vi "Autonomous Independent.vi"() -> ()   [LabVIEW 2016]
doc: "This VI is called when autonomous begins, and will automatically be terminated when autonomous ends. You can carry out timed or sensor driven robot movement independently without needing to return to the caller."
uses:
  2_8_17/Auto_Action.ctl
  <vilib>/Rock Robotics/Network Tables/NT Read Number.vi
  2_11_17/Systems/Global 1.vi
panel:
  out "Auto Mode":dbl=7.0
  in  "Auton_Modes":T2(array[cluster])=[{"Actions"=[{"Effort"=0.55, "Duration"=3.5, "Action"=enum."Nothing", "Encoder"=0.0, "Condition"=FALSE}, {"Effort"=0.0, "Duration"=0.0, "Action"=enum."Nothing", "Encoder"=0.0, "Condition"=FALSE}]}, {"Actions"=[{"Effort"=0.0, "Duration"=0.1, "Action"=enum."Gear1", "Encoder"=6.462, "Condition"=FALSE}, {"Effort"=0.0, "Duration"=0.1, "Action"=enum."Nothing", "Encoder"=0.0, "Condition"=FALSE}, {"Effort"=0.25, "Duration"=1.0, "Action"=enum."Nothing", "Encoder"=38.0, "Condition"=FALSE}, {"Effort"=0.0, "Duration"=0.1, "Action"=enum."Nothing", "Encoder"=0.0, "Condition"=FALSE}, {"Effort"=0.25, "Duration"=0.0, "Action"=enum."Nothing", "Encoder"=57.0, "Condition"=FALSE}, {"Effort"=-0.25, "Duration"=0.0, "Action"=enum."Nothing", "Encoder"=0.0, "Condition"=FALSE}, {"Effort"=1.0, "Duration"=0.0, "Action"=enum."Nothing", "Encoder"=0.0, "Condition"=FALSE}, {"Effort"=0.25, "Duration"=0.0, "Action"=enum."Nothing", "Encoder"=0.0, "Condition"=FALSE}]}, {"Actions"=[{"Effort"=0.0, "Duration"=0.1, "Action"=enum."Drive Encoder Reset", "Encoder"=0.0, "Condition"=FALSE}, {"Effort"=0.0, "Duration"=1.0, "Action"=enum."Gyro Reset", "Encoder"=0.0, "Condition"=FALSE}, {"Effort"=0.3, "Duration"=2.0, "Action"=enum."Drive", "Encoder"=88.0, "Condition"=TRUE}, {"Effort"=1.0, "Duration"=1.0, "Action"=enum."Gear0", "Encoder"=0.0, "Condition"=FALSE}, {"Effort"=1.0, "Duration"=1.0, "Action"=enum."Gear0", "Encoder"=0.0, "Condition"=FALSE}, {"Effort"=1.0, "Duration"=0.5, "Action"=enum."Nothing", "Encoder"=0.0, "Condition"=FALSE}, {"Effort"=0.0, "Duration"=0.0, "Action"=enum."Drive Encoder Reset", "Encoder"=0.0, "Condition"=FALSE}, {"Effort"=0.3, "Duration"=0.5, "Action"=enum."Nothing", "Encoder"=24.0, "Condition"=TRUE}, {"Effort"=0.0, "Duration"=0.0, "Action"=enum."Nothing", "Encoder"=0.0, "Condition"=FALSE}, {"Effort"=-0.2, "Duration"=0.75, "Action"=enum."Drive", "Encoder"=24.0, "Condition"=FALSE}, {"Effort"=0.0, "Duration"=0.0, "Action"=enum."Drive Encoder Reset", "Encoder"=0.0, "Condition"=FALSE}, {"Effort"=-0.25, "Duration"=0.0, "Action"=enum."Nothing", "Encoder"=12.0, "Condition"=FALSE}]}, {"Actions"=[{"Effort"=0.0, "Duration"=0.1, "Action"=enum."Drive Encoder Reset", "Encoder"=6.462, "Condition"=FALSE}, {"Effort"=0.0, "Duration"=0.1, "Action"=enum."Gyro Reset", "Encoder"=0.0, "Condition"=FALSE}, {"Effort"=-0.25, "Duration"=1.0, "Action"=enum."Drive", "Encoder"=6.462, "Condition"=FALSE}, {"Effort"=0.0, "Duration"=0.1, "Action"=enum."Gyro Reset", "Encoder"=0.0, "Condition"=FALSE}, {"Effort"=-0.25, "Duration"=0.0, "Action"=enum."Turn", "Encoder"=57.0, "Condition"=FALSE}, {"Effort"=-0.25, "Duration"=0.0, "Action"=enum."Drive", "Encoder"=7.5, "Condition"=FALSE}, {"Effort"=-1.0, "Duration"=0.0, "Action"=enum."Gear0", "Encoder"=0.0, "Condition"=FALSE}, {"Effort"=0.25, "Duration"=0.0, "Action"=enum."Drive", "Encoder"=3.0, "Condition"=FALSE}]}, {"Actions"=[{"Effort"=0.0, "Duration"=0.1, "Action"=enum."Drive Encoder Reset", "Encoder"=6.462, "Condition"=FALSE}, {"Effort"=0.0, "Duration"=0.1, "Action"=enum."Gyro Reset", "Encoder"=0.0, "Condition"=FALSE}, {"Effort"=-0.25, "Duration"=1.0, "Action"=enum."Drive", "Encoder"=6.462, "Condition"=FALSE}, {"Effort"=0.0, "Duration"=0.1, "Action"=enum."Gyro Reset", "Encoder"=0.0, "Condition"=FALSE}, {"Effort"=-0.25, "Duration"=0.0, "Action"=enum."Turn", "Encoder"=57.0, "Condition"=FALSE}, {"Effort"=-0.25, "Duration"=0.0, "Action"=enum."Drive", "Encoder"=7.5, "Condition"=FALSE}, {"Effort"=-1.0, "Duration"=0.0, "Action"=enum."Gear0", "Encoder"=0.0, "Condition"=FALSE}, {"Effort"=0.25, "Duration"=0.0, "Action"=enum."Drive", "Encoder"=3.0, "Condition"=FALSE}]}, {"Actions"=[{"Effort"=0.0, "Duration"=0.1, "Action"=enum."Drive Encoder Reset", "Encoder"=0.0, "Condition"=FALSE}, {"Effort"=0.0, "Duration"=0.1, "Action"=enum."Gyro Reset", "Encoder"=0.0, "Condition"=FALSE}, {"Effort"=0.25, "Duration"=1.0, "Action"=enum."Drive", "Encoder"=6.462, "Condition"=FALSE}, {"Effort"=1.0, "Duration"=0.1, "Action"=enum."Gyro Reset", "Encoder"=0.0, "Condition"=FALSE}, {"Effort"=0.25, "Duration"=0.0, "Action"=enum."Turn", "Encoder"=57.0, "Condition"=FALSE}, {"Effort"=0.25, "Duration"=0.0, "Action"=enum."Drive", "Encoder"=7.5, "Condition"=FALSE}, {"Effort"=1.0, "Duration"=0.0, "Action"=enum."Gear0", "Encoder"=0.0, "Condition"=FALSE}, {"Effort"=-0.25, "Duration"=0.0, "Action"=enum."Drive", "Encoder"=3.0, "Condition"=FALSE}]}, {"Actions"=[{"Effort"=0.0, "Duration"=0.1, "Action"=enum."Drive Encoder Reset", "Encoder"=0.0, "Condition"=FALSE}, {"Effort"=0.0, "Duration"=0.1, "Action"=enum."Gyro Reset", "Encoder"=0.0, "Condition"=FALSE}, {"Effort"=0.25, "Duration"=5.0, "Action"=enum."Drive", "Encoder"=60000.0, "Condition"=TRUE}, {"Effort"=0.75, "Duration"=1.0, "Action"=enum."Nothing", "Encoder"=0.0, "Condition"=FALSE}, {"Effort"=0.0, "Duration"=1.0, "Action"=enum."Nothing", "Encoder"=0.0, "Condition"=FALSE}, {"Effort"=0.0, "Duration"=0.0, "Action"=enum."Nothing", "Encoder"=0.0, "Condition"=FALSE}]}, {"Actions"=[{"Effort"=0.0, "Duration"=0.5, "Action"=enum."Drive Encoder Reset", "Encoder"=0.0, "Condition"=FALSE}, {"Effort"=0.55, "Duration"=4.25, "Action"=enum."Gyro Reset", "Encoder"=0.0, "Condition"=FALSE}, {"Effort"=0.3, "Duration"=0.0, "Action"=enum."Drive", "Encoder"=60.0, "Condition"=FALSE}, {"Effort"=0.25, "Duration"=1.5, "Action"=enum."Turn", "Encoder"=0.0, "Condition"=FALSE}, {"Effort"=0.25, "Duration"=2.0, "Action"=enum."Vision Correction", "Encoder"=76.6, "Condition"=FALSE}, {"Effort"=0.3, "Duration"=0.5, "Action"=enum."Drive", "Encoder"=0.0, "Condition"=TRUE}]}, {"Actions"=[{"Effort"=0.0, "Duration"=0.0, "Action"=enum."Nothing", "Encoder"=0.0, "Condition"=FALSE}]}]
  # "Nothing"
  # "Boiler Right Right side gear"
  # "Middle Gear"
  # "Boiler Right Left Side Gear"
  # "Boiler Left RightSide Gear"
  # "Boiler Left Left Side Gear"
  # "Drive"
  # "Vision Correction"
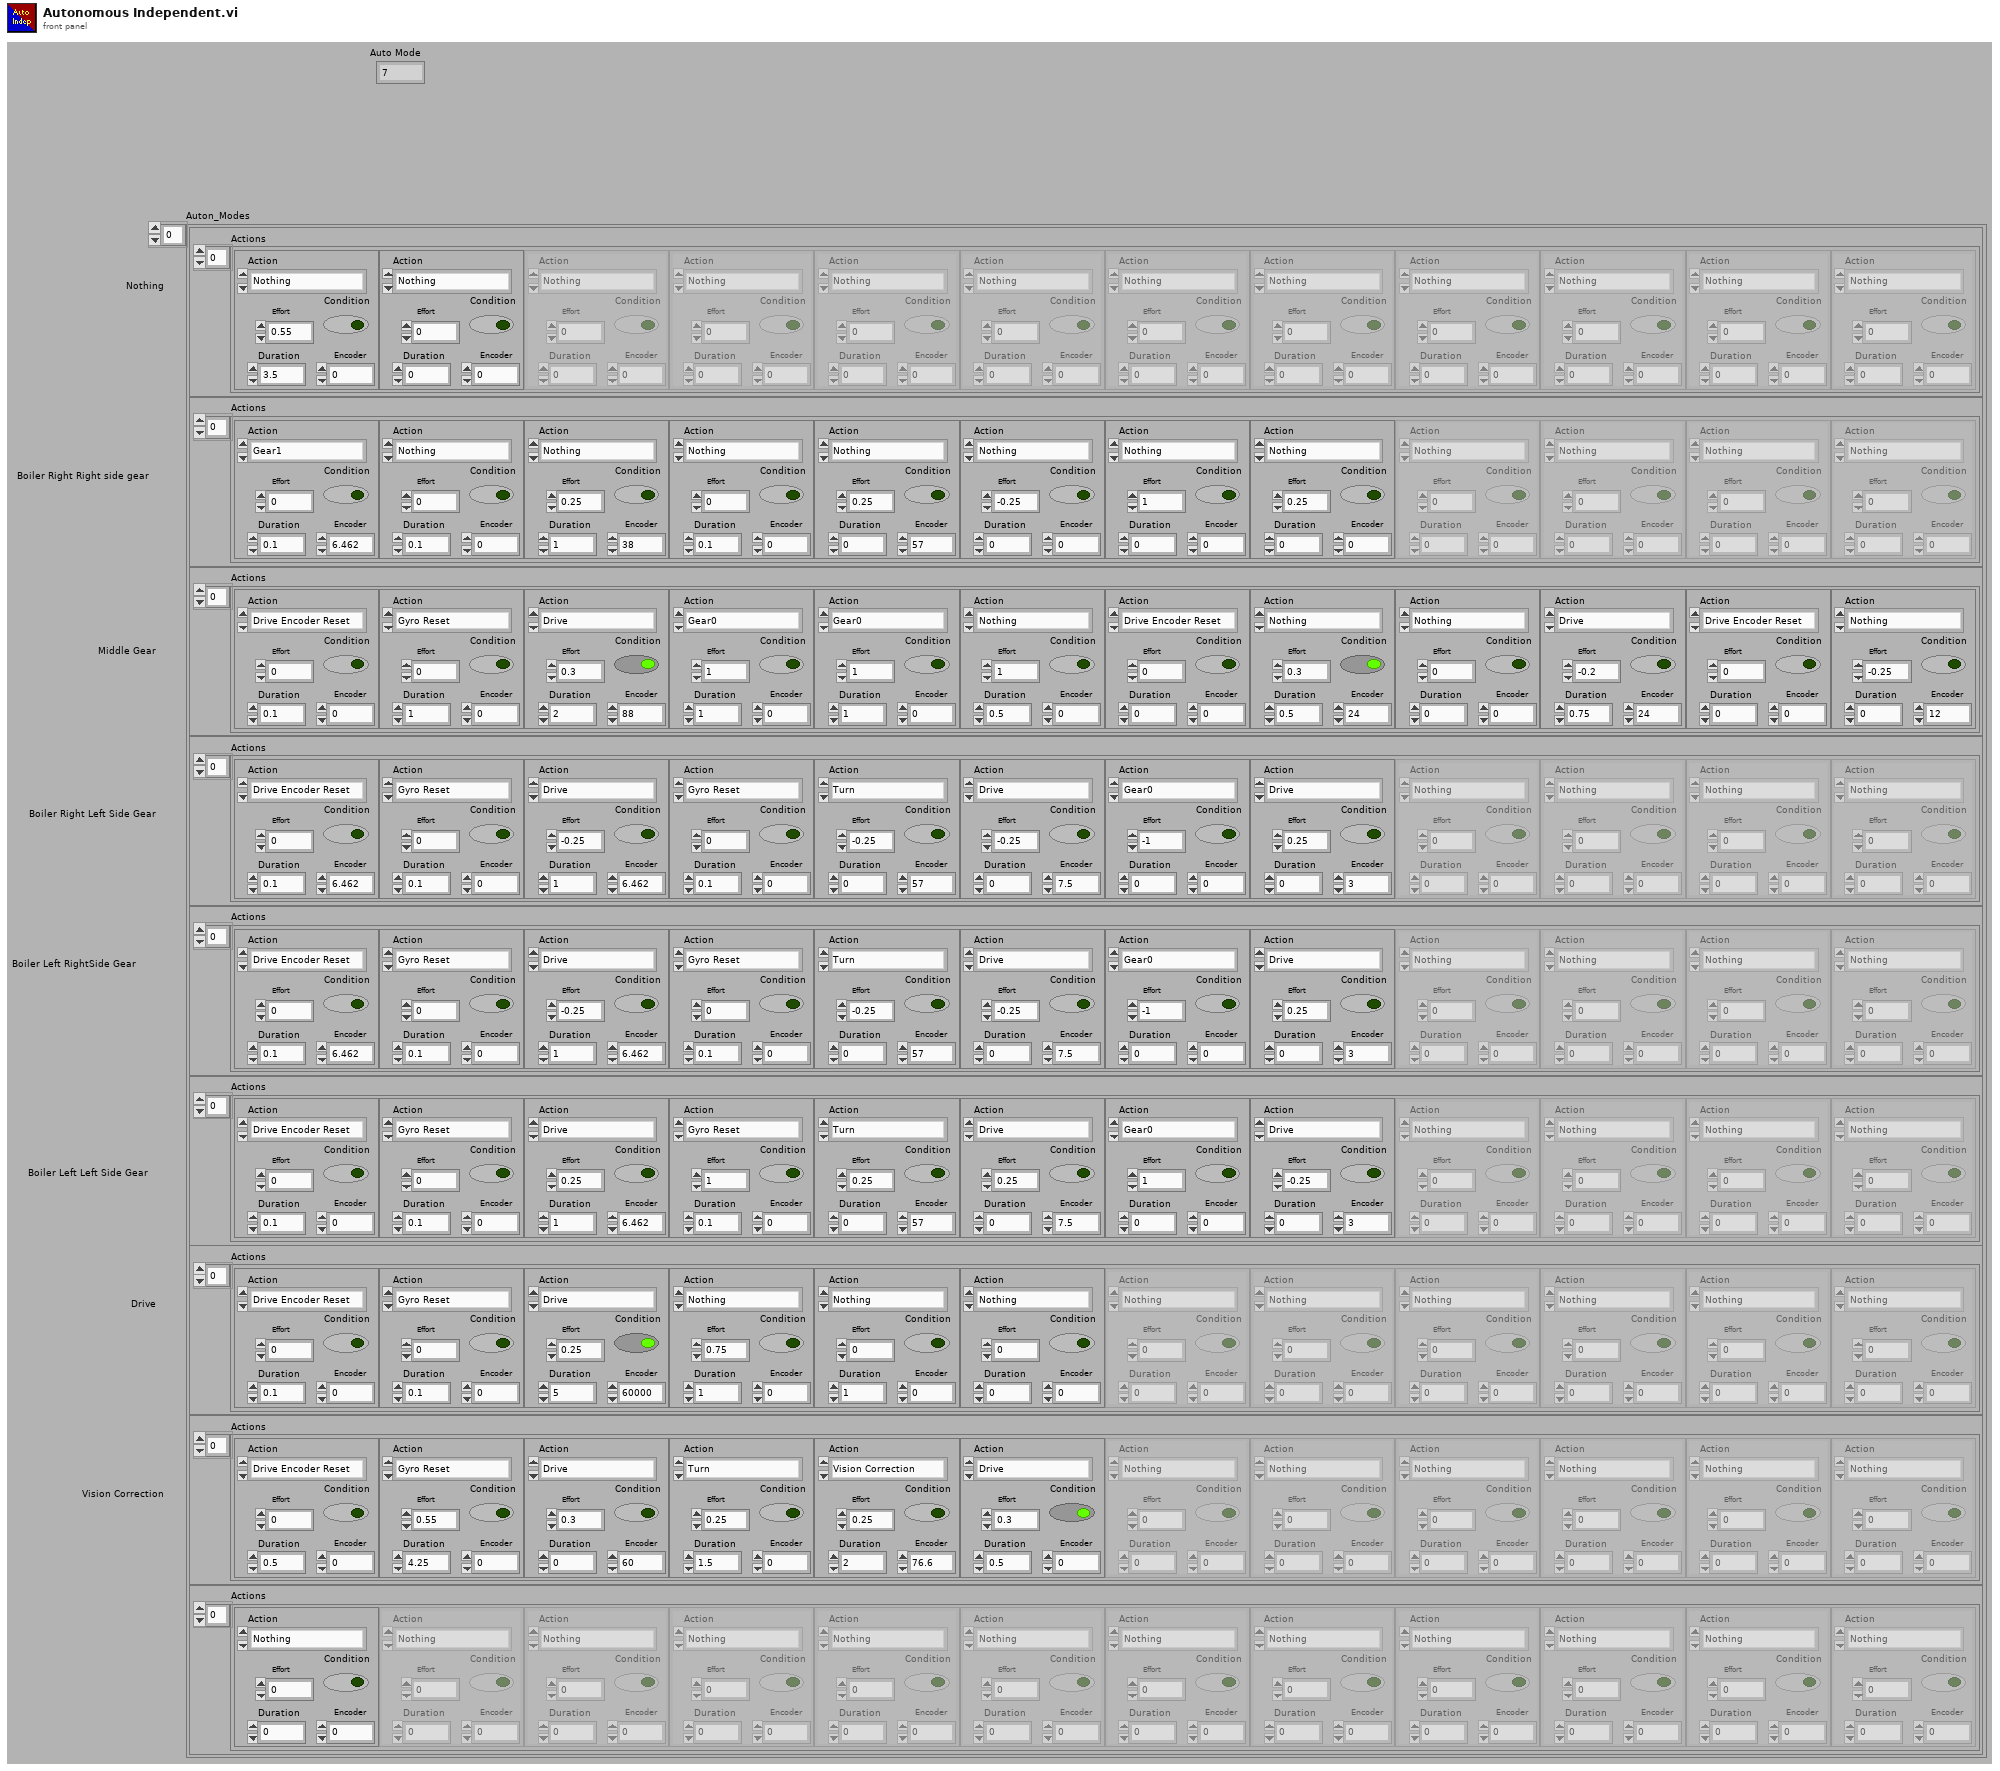
[diagram p1: front panel]
types:
  T1 = typedef "Auto_Action.ctl" = enum16{"Nothing", "Drive", "Vision Correction", "Turn", "Gear0", "Gear1", "Climb", "Intake", "Index", "Shoot", "Test", "Drive Encoder Reset", "Gyro Reset"}
  T2 = cluster{"Actions":cluster{"Effort":dbl, "Duration":dbl, "Action":T1, "Encoder":dbl, "Condition":bool}[]}[]
  T3 = cluster{"Actions":cluster{"Effort":dbl, "Duration":dbl, "Action":T1, "Encoder":dbl, "Condition":bool}[]}
  T4 = cluster{"Effort":dbl, "Duration":dbl, "Action":T1, "Encoder":dbl, "Condition":bool}[]
  T5 = typedef "WPI_MotorControlDeviceRef.ctl" = cluster{"DeviceStatus":errorcluster, "Type":T6, "PWM":cluster{"PWM Channel":T7, "DeadBand":T8}, "CAN":cluster{"Device Number":u8, "SetOutput VI Ref":variant, "GetOutput VI Ref":variant, "Enable VI Ref":variant, "Disable VI Ref":variant, "Data":variant}, "Invert":bool}
  T6 = typedef "WPI_MotorControlType.ctl" = enum16{"PWM", "CAN"}
  T7 = typedef "FPGA_DIOPWMChannel.ctl" = enum8{"PWM 0", "PWM 1", "PWM 2", "PWM 3", "PWM 4", "PWM 5", "PWM 6", "PWM 7", "PWM 8", "PWM 9", "PWM MXP 0", "PWM MXP 1", "PWM MXP 2", "PWM MXP 3", "PWM MXP 4", "PWM MXP 5", "PWM MXP 6", "PWM MXP 7", "PWM MXP 8", "PWM MXP 9", "Invalid"}
  T8 = typedef "WPI_PWMDeadband.ctl" = cluster{"Name":string, "maxPositivePwm":i32, "minPositivePwm":i32, "centerPwm":i32, "maxNegativePwm":i32, "minNegativePwm":i32, "angularRange":u16}
  T9 = typedef "WPI_CANTalonSRX_GlobalStatus.ctl" = cluster{"Applied Throttle":dbl, "Module Enabled":bool, "CAN Error":errorcluster, "Closed Loop Error":dbl, "Forward Limit Switch Closed":bool, "Reverse Limit Switch Closed":bool, "Sensor Position":dbl, "Sensor Velocity":dbl, "Current":dbl, "Sticky Fault - Over Temp":bool, "Sticky Fault - Under Voltage":bool, "Sticky Fault - Forward Limit":bool, "Sticky Fault - Reverse Limit":bool, "Sticky Fault - Forward Soft Limit":bool, "Sticky Fault - Reverse Soft Limit":bool, "Brake is Enabled":bool, "Encoder Position":dbl, "Encoder Velocity":dbl, "Encoder Index Count":dbl, "Encoder A Pin State":bool, "Encoder B Pin State":bool, "Encoder Index Pin State":bool, "Analog In":dbl, "Analog In Velocity":dbl, "Temperature (C)":dbl, "Battery Voltage":dbl, "Control 5 Is Supported":bool, "Current Profile Slot Select":dbl, "Pos Div 8":bool, "Vel Div 4":bool, "Pulse Width Position":i32, "Pulse Width Velocity":i32, "Pulse Width Rise To Rise (us)":i32, "Pulse Width Rise To Fall (us)":i32, "Mot Prof Active Is Under Run":bool, "Mot Prof Active Has Under Run":bool, "Mot Prof Active Is Last":bool, "Mot Prof Active Velocity Only":bool, "Mot Prof Active Is Valid":bool, "Mot Prof Buffer Is Full":bool, "Mot Prof Active Profile Slot Select":i32, "Mot Prof NextID":i32, "Mot Prof Count":i32, "Mot Prof Active Velocity":dbl, "Mot Prof Active Position":dbl, "Mot Prof Output Enable":i32}
  T10 = typedef "WPI_GyroDevRef.ctl" = cluster{"DevStatus":errorcluster, "Analog Channel":T11, "Offset":dbl, "Gain (VoltsPerDegree/Second)":dbl, "Gyro Type":enum16{"Analog", "XRS450"}, "Handle":i32, "SPI Bus":T12, "Device Found":bool, "Sample Rate":dbl, "Calibrate On Open":bool}
  T11 = typedef "FPGA_AIChannel.ctl" = enum8{"AI 0", "AI 1", "AI 2", "AI 3", "AI MXP 0", "AI MXP 1", "AI MXP 2", "AI MXP 3", "Invalid"}
  T12 = typedef "spi_bus.ctl" = enum16{"SPI On-Board, CS0", "SPI On-Board, CS1", "SPI On-Board, CS2", "SPI On-Board, CS3", "SPI MXP", "Invalid"}
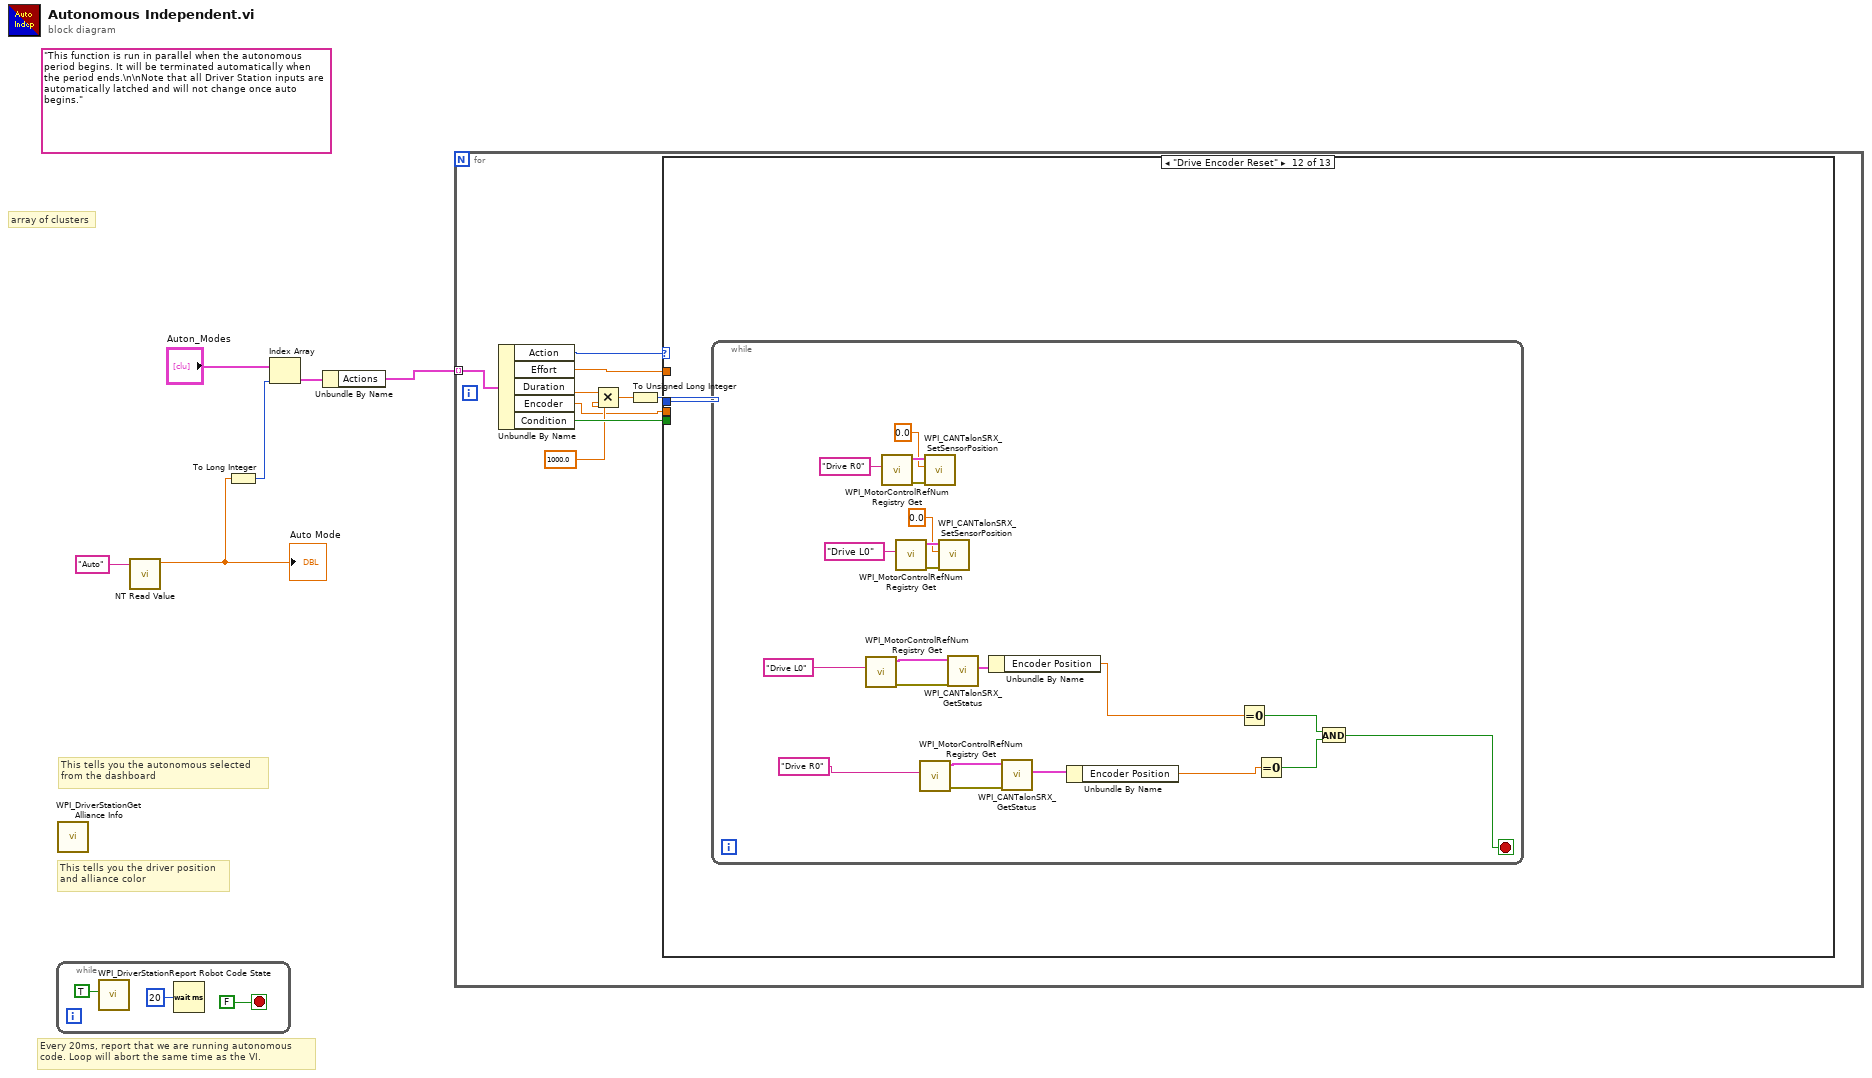
[diagram p0: block diagram]
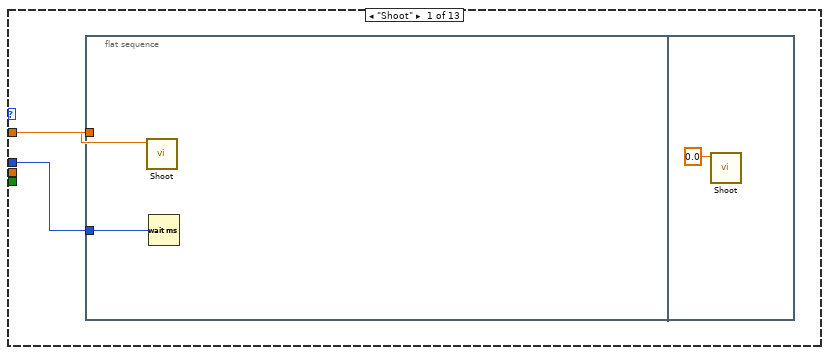
[diagram p2: hidden frame]
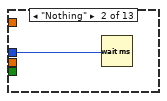
[diagram p3: hidden frame]
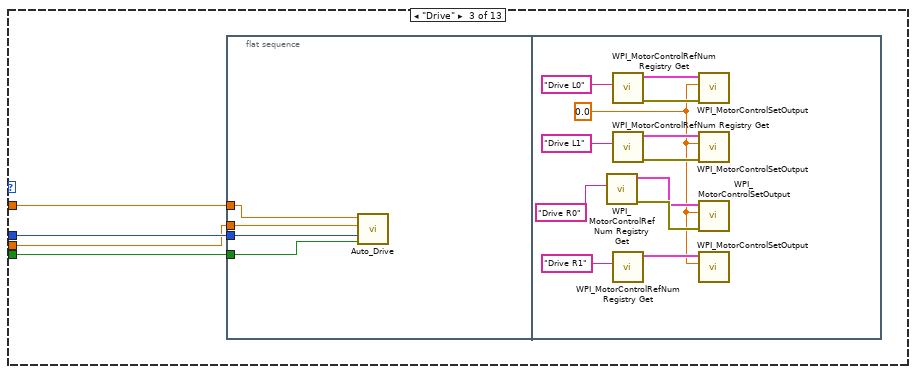
[diagram p4: hidden frame]
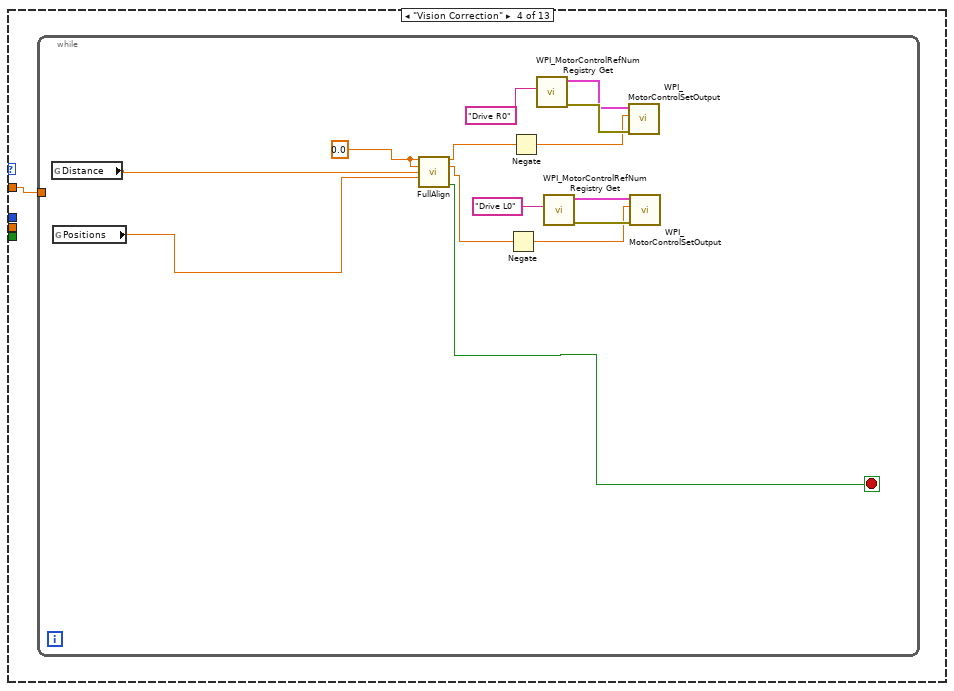
[diagram p5: hidden frame]
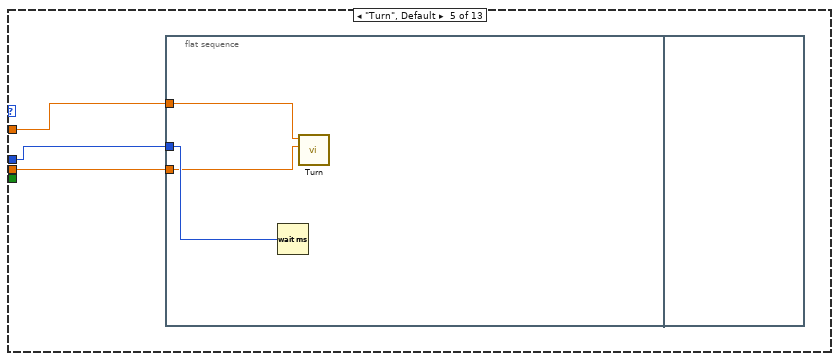
[diagram p6: hidden frame]
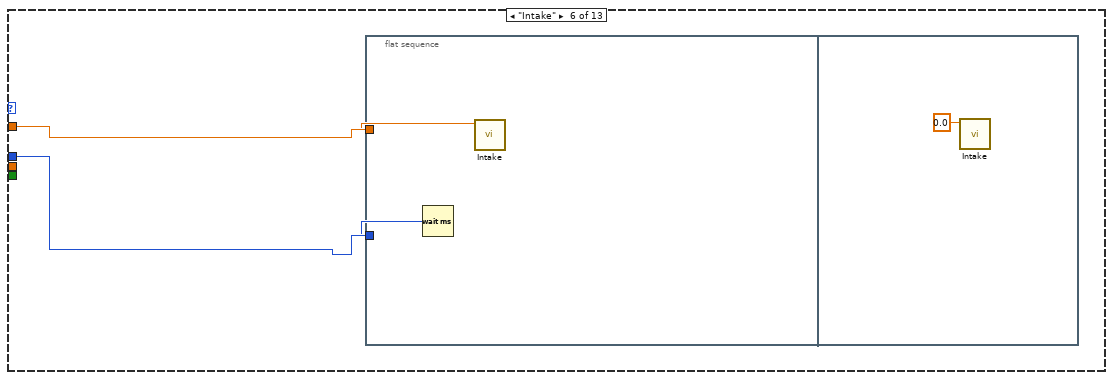
[diagram p7: hidden frame]
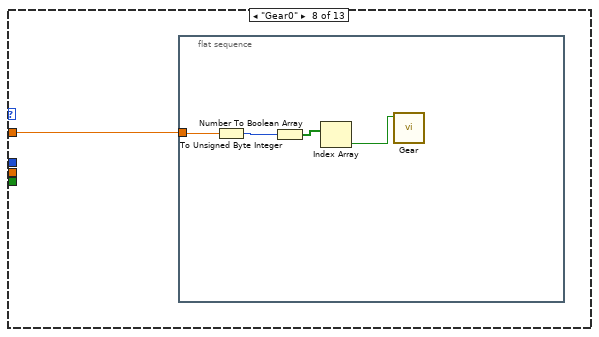
[diagram p9: hidden frame]
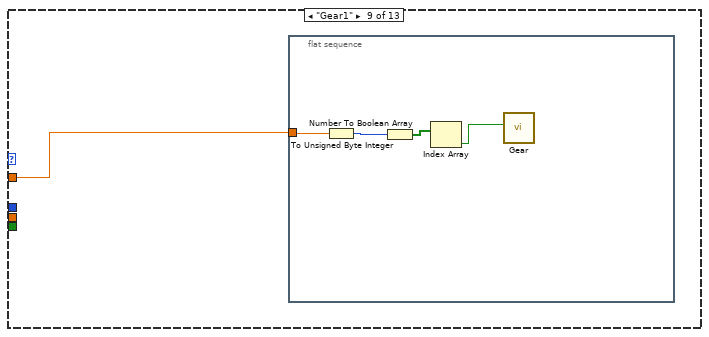
[diagram p10: hidden frame]
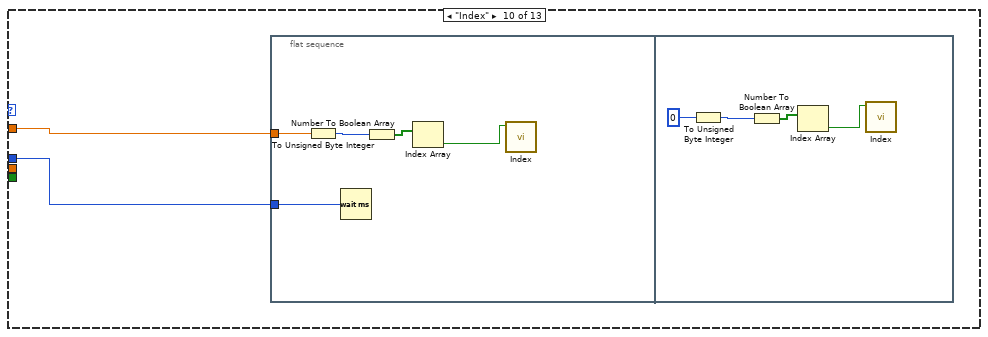
[diagram p11: hidden frame]
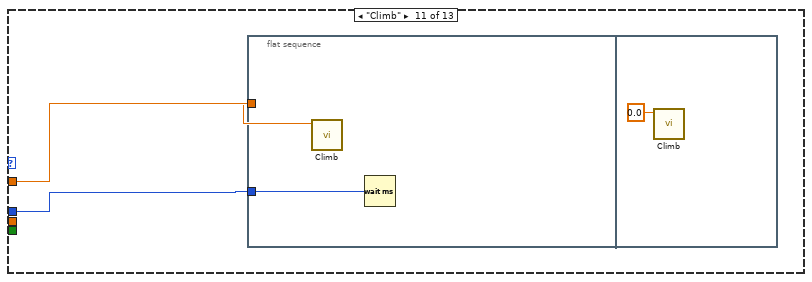
[diagram p12: hidden frame]
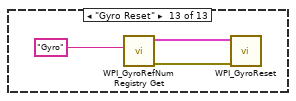
[diagram p13: hidden frame]
diagram:
  (unwired) "This function is run in parallel when the autonomous period begins. It will be terminated automatically when the period ends.\n\nNote that all Driver Station inputs are automatically latched and will not change once auto begins."
  # "This tells you the autonomous selected\nfrom the dashboard"
  # "array of clusters"
  # "Every 20ms, report that we are running autonomous\ncode. Loop will abort the same time as the VI."
  # "This tells you the driver position\nand alliance color"
  n1 = while {
    stop <- FALSE stop-if-true
    n2 = call <vilib>:"WPI_DriverStationReport Robot Code State.vi"("Autonomous"=TRUE) -> ()  [unwired: 10 in, 1 out]
    n3 = Wait (ms)(milliseconds to wait=u32 20) -> ()  [unwired: 1 out]
  }
  n4 = call <vilib>:"WPI_DriverStationGet Alliance Info.vi"() -> ()  [unwired: 12 out]
  n5 = call-poly <vilib>:"NT Read Value.vi"("Name"="Auto") -> ("Numeric"=w1:dbl)  [unwired: 9 in, 1 out]
  "Auto Mode" <- w1
  n6 = To Long Integer(number=w1) -> (32bit integer=w3:i32)
  n7 = Index Array(array="Auton_Modes", index=w3) -> (element=w5:T3)
  n8 = Unbundle By Name(w5) -> ("Actions"=w6:T4)
  n9 = for {
    tunnel: w6 -> [w18] mode=indexing
    n10 = Unbundle By Name(w18) -> ("Action"=w17:T1, "Effort"=w16:dbl, "Duration"=w15:dbl, "Encoder"=w10:dbl, "Condition"=w12:bool)
    n11 = Multiply(x=w15, y=1000.0) -> (x*y=w14:dbl)
    n12 = To Unsigned Long Integer(number=w14) -> (unsigned 32bit integer=w13:u32)
    n13 = case shown="\"Drive Encoder Reset\"" w17 {
      tunnel: w16 -> [w20 _ w28 w45 w62 w67 _ w71 w76 w81 w93 _ _]
      tunnel: w13 -> [w19 w24 w27 _ w61 w66 _ _ _ w82 w92 _ _]
      tunnel: w12 -> [_ _ w26 _ _ _ _ _ _ _ _ _ _]
      tunnel: w10 -> [_ _ w25 _ w60 _ _ _ _ _ _ _ _]
      frame "Shoot" {
        n14 = flat-sequence {
          tunnel: w20 -> [w22]
          tunnel: w19 -> [w21]
          frame #0 {
            n15 = call "Shoot.vi"("Set RPM"=w22) -> ()  [unwired: 11 in]
            n16 = Wait (ms)(milliseconds to wait=w21) -> ()  [unwired: 1 out]
          }
          frame #1 {
            n17 = call "Shoot.vi"("Set RPM"=0.0 ("Effort")) -> ()  [unwired: 11 in]
          }
        }
      }
      frame "Nothing" {
        n18 = Wait (ms)(milliseconds to wait=w24) -> ()  [unwired: 1 out]
      }
      frame "Drive" {
        n19 = flat-sequence {
          tunnel: w28 -> [w32]
          tunnel: w27 -> [w31]
          tunnel: w26 -> [w30]
          tunnel: w25 -> [w29]
          frame #0 {
            n20 = call "Auto_Drive.vi"("Timer?"=w30, "Duration"=w31, "distance"=w29, "Drive Effort"=w32) -> ()  [unwired: 8 in]
          }
          frame #1 {
            w33 = 0.0 ("Drive L")
            n21 = call <vilib>:"WPI_MotorControlRefNum Registry Get.vi"("refnum name"="Drive R0") -> ("error out"=w38:errorcluster, "MotorControlDevRef"=w34:T5)  [unwired: 9 in]
            n22 = call <vilib>:"WPI_MotorControlRefNum Registry Get.vi"("refnum name"="Drive L0") -> ("error out"=w39:errorcluster, "MotorControlDevRef"=w40:T5)  [unwired: 9 in]
            n23 = call <vilib>:"WPI_MotorControlRefNum Registry Get.vi"("refnum name"="Drive L1") -> ("error out"=w43:errorcluster, "MotorControlDevRef"=w42:T5)  [unwired: 9 in]
            n24 = call <vilib>:"WPI_MotorControlRefNum Registry Get.vi"("refnum name"="Drive R1") -> ("MotorControlDevRef"=w36:T5)  [unwired: 9 in, 1 out]
            n25 = call <vilib>:"WPI_MotorControlSetOutput.vi"("error in (no error)"=w39, "Output"=w33, "MotorControlDevRef"=w40) -> ()  [unwired: 6 in, 3 out]
            n26 = call <vilib>:"WPI_MotorControlSetOutput.vi"("error in (no error)"=w43, "Output"=w33, "MotorControlDevRef"=w42) -> ()  [unwired: 6 in, 3 out]
            n27 = call <vilib>:"WPI_MotorControlSetOutput.vi"("error in (no error)"=w38, "Output"=w33, "MotorControlDevRef"=w34) -> ()  [unwired: 6 in, 3 out]
            n28 = call <vilib>:"WPI_MotorControlSetOutput.vi"("Output"=w33, "MotorControlDevRef"=w36) -> ()  [unwired: 7 in, 3 out]
          }
        }
      }
      frame "Vision Correction" {
        n29 = while {
          tunnel: w45 -> [_]
          stop <- w50 stop-if-true
          w53 = 0.0
          n30 = global read "Global 1.vi" "Distance"() -> (w52:dbl)
          n31 = global read "Global 1.vi" "Positions"() -> (w51:dbl)
          n32 = call "FullAlign.vi"("Joystick 0"=w53, "Joystick 1"=w53, "Distance"=w52, "Angle"=w51) -> ("Right Motor"=w48:dbl, "Left Motor"=w49:dbl, "In Range?"=w50:bool)  [unwired: 9 in]
          n33 = Negate(x=w49) -> (-x=w46:dbl)
          n34 = Negate(x=w48) -> (-x=w47:dbl)
          n35 = call <vilib>:"WPI_MotorControlRefNum Registry Get.vi"("refnum name"="Drive R0") -> ("error out"=w56:errorcluster, "MotorControlDevRef"=w54:T5)  [unwired: 9 in]
          n36 = call <vilib>:"WPI_MotorControlRefNum Registry Get.vi"("refnum name"="Drive L0") -> ("error out"=w57:errorcluster, "MotorControlDevRef"=w58:T5)  [unwired: 9 in]
          n37 = call <vilib>:"WPI_MotorControlSetOutput.vi"("error in (no error)"=w56, "Output"=w47, "MotorControlDevRef"=w54) -> ()  [unwired: 6 in, 3 out]
          n38 = call <vilib>:"WPI_MotorControlSetOutput.vi"("error in (no error)"=w57, "Output"=w46, "MotorControlDevRef"=w58) -> ()  [unwired: 6 in, 3 out]
        }
      }
      frame "Turn", Default {
        n39 = flat-sequence {
          tunnel: w62 -> [w65]
          tunnel: w61 -> [w64]
          tunnel: w60 -> [w63]
          frame #0 {
            n40 = Wait (ms)(milliseconds to wait=w64) -> ()  [unwired: 1 out]
            n41 = call "Turn.vi"("Target"=w63, "Effort"=w65) -> ()  [unwired: 10 in]
          }
          frame #1 {
          }
        }
      }
      frame "Intake" {
        n42 = flat-sequence {
          tunnel: w67 -> [w69]
          tunnel: w66 -> [w68]
          frame #0 {
            n43 = Wait (ms)(milliseconds to wait=w68) -> ()  [unwired: 1 out]
            n44 = call "Intake.vi"("Effort"=w69) -> ()  [unwired: 11 in]
          }
          frame #1 {
            n45 = call "Intake.vi"("Effort"=0.0) -> ()  [unwired: 11 in]
          }
        }
      }
      frame "Test" {
      }
      frame "Gear0" {
        n46 = flat-sequence {
          tunnel: w71 -> [w75]
          frame #0 {
            n47 = To Unsigned Byte Integer(number=w75) -> (unsigned 8bit integer=w74:u8)
            n48 = Number To Boolean Array(number=w74) -> (Boolean array=w73:bool[])
            n49 = Index Array(array=w73) -> (element=w72:bool)  [unwired: 1 in]
            n50 = call "Gear.vi"("Gear0?"=w72) -> ()  [unwired: 11 in]
          }
        }
      }
      frame "Gear1" {
        n51 = flat-sequence {
          tunnel: w76 -> [w80]
          frame #0 {
            n52 = To Unsigned Byte Integer(number=w80) -> (unsigned 8bit integer=w79:u8)
            n53 = Number To Boolean Array(number=w79) -> (Boolean array=w78:bool[])
            n54 = Index Array(array=w78) -> (element=w77:bool)  [unwired: 1 in]
            n55 = call "Gear.vi"("Gear1?"=w77) -> ()  [unwired: 11 in]
          }
        }
      }
      frame "Index" {
        n56 = flat-sequence {
          tunnel: w82 -> [w84]
          tunnel: w81 -> [w83]
          frame #0 {
            n57 = To Unsigned Byte Integer(number=w83) -> (unsigned 8bit integer=w87:u8)
            n58 = Wait (ms)(milliseconds to wait=w84) -> ()  [unwired: 1 out]
            n59 = Number To Boolean Array(number=w87) -> (Boolean array=w86:bool[])
            n60 = Index Array(array=w86) -> (element=w85:bool)  [unwired: 1 in]
            n61 = call "Index.vi"("Index?"=w85) -> ()  [unwired: 11 in]
          }
          frame #1 {
            n62 = To Unsigned Byte Integer(number=u8 0) -> (unsigned 8bit integer=w90:u8)
            n63 = Number To Boolean Array(number=w90) -> (Boolean array=w91:bool[])
            n64 = Index Array(array=w91) -> (element=w88:bool)  [unwired: 1 in]
            n65 = call "Index.vi"("Index?"=w88) -> ()  [unwired: 11 in]
          }
        }
      }
      frame "Climb" {
        n66 = flat-sequence {
          tunnel: w93 -> [w95]
          tunnel: w92 -> [w94]
          frame #0 {
            n67 = call "Climb.vi"("Effort"=w95) -> ()  [unwired: 11 in]
            n68 = Wait (ms)(milliseconds to wait=w94) -> ()  [unwired: 1 out]
          }
          frame #1 {
            n69 = call "Climb.vi"("Effort"=0.0) -> ()  [unwired: 11 in]
          }
        }
      }
      frame "Drive Encoder Reset" {
        n70 = while {
          stop <- w97 stop-if-true
          n71 = call <vilib>:"WPI_MotorControlRefNum Registry Get.vi"("refnum name"="Drive L0") -> ("error out"=w107:errorcluster, "MotorControlDevRef"=w102:T5)  [unwired: 9 in]
          n72 = call <vilib>:"WPI_MotorControlRefNum Registry Get.vi"("refnum name"="Drive R0") -> ("error out"=w112:errorcluster, "MotorControlDevRef"=w111:T5)  [unwired: 9 in]
          n73 = call <vilib>:"WPI_MotorControlRefNum Registry Get.vi"("refnum name"="Drive L0") -> ("error out"=w114:errorcluster, "MotorControlDevRef"=w115:T5)  [unwired: 9 in]
          n74 = call <vilib>:"WPI_MotorControlRefNum Registry Get.vi"("refnum name"="Drive R0") -> ("error out"=w104:errorcluster, "MotorControlDevRef"=w103:T5)  [unwired: 9 in]
          n75 = call <vilib>:"WPI_CANTalonSRX_SetSensorPosition.vi"("error in (no error)"=w112, "New Sensor Position"=0.0, "CAN Talon SRX Ref"=w111) -> ()  [unwired: 7 in, 2 out]
          n76 = call <vilib>:"WPI_CANTalonSRX_SetSensorPosition.vi"("error in (no error)"=w114, "New Sensor Position"=0.0, "CAN Talon SRX Ref"=w115) -> ()  [unwired: 7 in, 2 out]
          n77 = call <vilib>:"WPI_CANTalonSRX_GetStatus.vi"("error in (no error)"=w107, "CAN Talon SRX Ref"=w102) -> ("Talon SRX Status"=w105:T9)  [unwired: 7 in, 2 out]
          n78 = Unbundle By Name(w105) -> ("Encoder Position"=w100:dbl)
          n79 = call <vilib>:"WPI_CANTalonSRX_GetStatus.vi"("error in (no error)"=w104, "CAN Talon SRX Ref"=w103) -> ("Talon SRX Status"=w106:T9)  [unwired: 7 in, 2 out]
          n80 = Unbundle By Name(w106) -> ("Encoder Position"=w101:dbl)
          n81 = Equal To 0?(x=w100) -> (x = 0?=w99:bool)
          n82 = Equal To 0?(x=w101) -> (x = 0?=w98:bool)
          n83 = And(x=w99, y=w98) -> (x .and. y?=w97:bool)
        }
      }
      frame "Gyro Reset" {
        n84 = call <vilib>:"WPI_GyroRefNum Registry Get.vi"("refnum name"="Gyro") -> ("error out"=w119:errorcluster, "GyroDevRef"=w120:T10)  [unwired: 9 in]
        n85 = call <vilib>:"WPI_GyroReset.vi"("error in"=w119, "GyroDevRef"=w120) -> ()  [unwired: 8 in, 2 out]
      }
    }
  }
